vi "RSZVB Start Fixture Compensation Sweep.vi"(8 "error in (no error)":errorcluster {"code" format="%.0x"}, 10 "Channel (1)":i32=1, 11 "VISA session":refnum<visa-resource-name>) -> (0 "error out":errorcluster {"code" format="%.0x"}, 3 "dup VISA session":refnum<visa-resource-name>)   [LabVIEW 2011]
doc: "Prepares the analyzer for fixture compensation comprising a single or a series of fixture compensation sweeps. Previous compensation data is deleted.\n\nRemote-control command(s):\n[SENSe<Ch>:]CORRection:COLLect:FIXTure:STARt"
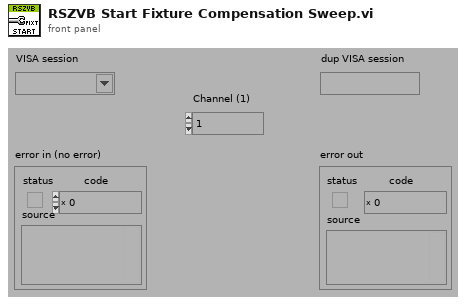
[diagram p1: front panel]
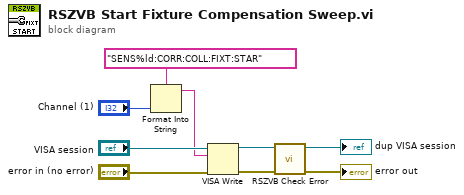
[diagram p0: block diagram]
diagram:
  n1 = Format Into String(format string="SENS%ld:CORR:COLL:FIXT:STAR", "Channel (1)") -> (resulting string=w5:string)  [unwired: 2 in, 1 out]
  n2 = VISA Write(VISA resource name="VISA session", write buffer=w5, error in (no error)="error in (no error)") -> (VISA resource name out=w3:refnum<visa-resource-name>, error out=w4:errorcluster)  [unwired: 1 out]
  n3 = call "RSZVB Check Error.vi"("error in (no error)"=w4, "VISA session"=w3) -> ("error out"=→"error out":errorcluster, "dup VISA session"=→"dup VISA session":refnum<visa-resource-name>)  [unwired: 8 in]
